vi "HFRR ADV v11.vi"() -> ()   [LabVIEW 2025] (continued)
        n1007 = property on="Imaging" class="Bool (strict)"("DisabledEnum"=w968) -> ()  [unwired: 2 in, 2 out]
        n1008 = property on="Analysis" class="Bool (strict)"("DisabledEnum"=w968) -> ()  [unwired: 2 in, 2 out]
        n1009 = property on="Home" class="Bool (strict)"("DisabledEnum"=w968) -> ()  [unwired: 2 in, 2 out]
        n1010 = property on="Report" class="Bool (strict)"("DisabledEnum"=w968) -> ()  [unwired: 2 in, 2 out]
        n1011 = property on="Test Setup" class="Bool (strict)"("DisabledEnum"=w968) -> ()  [unwired: 2 in, 2 out]
        n1012 = case shown="True" w967 {
          tunnel: [T16."Disabled" ("Disabled") T16."Enabled" ("Disabled")] -> w966
          frame False {
          }
          frame True {
          }
        }
        n1013 = property on="About" class="Bool (strict)"("DisabledEnum"=w966) -> ()  [unwired: 2 in, 2 out]
      }
      frame "Adv Scar" {
        w975 = T16."Enabled" ("Disabled")
        n1014 = property on="Dashboard" class="Bool (strict)"("DisabledEnum"=T16."Disabled" ("Disabled")) -> ()  [unwired: 2 in, 2 out]
        n1015 = property on="Imaging" class="Bool (strict)"("DisabledEnum"=w975) -> ()  [unwired: 2 in, 2 out]
        n1016 = property on="Analysis" class="Bool (strict)"("DisabledEnum"=w975) -> ()  [unwired: 2 in, 2 out]
        n1017 = property on="Home" class="Bool (strict)"("DisabledEnum"=w975) -> ()  [unwired: 2 in, 2 out]
        n1018 = property on="Report" class="Bool (strict)"("DisabledEnum"=w975) -> ()  [unwired: 2 in, 2 out]
        n1019 = property on="Test Setup" class="Bool (strict)"("DisabledEnum"=w975) -> ()  [unwired: 2 in, 2 out]
        n1020 = local read "Service Password enable"() -> (w973:bool)
        n1021 = case shown="True" w973 {
          tunnel: [T16."Disabled" ("Disabled") T16."Enabled" ("Disabled")] -> w972
          frame False {
          }
          frame True {
          }
        }
        n1022 = property on="About" class="Bool (strict)"("DisabledEnum"=w972) -> ()  [unwired: 2 in, 2 out]
      }
      frame "Adv Scar Report" {
        w980 = T16."Enabled" ("Disabled")
        n1023 = property on="Dashboard" class="Bool (strict)"("DisabledEnum"=T16."Disabled" ("Disabled")) -> ()  [unwired: 2 in, 2 out]
        n1024 = property on="Imaging" class="Bool (strict)"("DisabledEnum"=w980) -> ()  [unwired: 2 in, 2 out]
        n1025 = property on="Analysis" class="Bool (strict)"("DisabledEnum"=w980) -> ()  [unwired: 2 in, 2 out]
        n1026 = property on="Home" class="Bool (strict)"("DisabledEnum"=w980) -> ()  [unwired: 2 in, 2 out]
        n1027 = property on="Report" class="Bool (strict)"("DisabledEnum"=w980) -> ()  [unwired: 2 in, 2 out]
        n1028 = property on="Test Setup" class="Bool (strict)"("DisabledEnum"=w980) -> ()  [unwired: 2 in, 2 out]
        n1029 = local read "Service Password enable"() -> (w979:bool)
        n1030 = case shown="True" w979 {
          tunnel: [T16."Disabled" ("Disabled") T16."Enabled" ("Disabled")] -> w978
          frame False {
          }
          frame True {
          }
        }
        n1031 = property on="About" class="Bool (strict)"("DisabledEnum"=w978) -> ()  [unwired: 2 in, 2 out]
      }
      frame "Compare Files" {
        w986 = T16."Enabled" ("Disabled")
        n1032 = local read "Service Password enable"() -> (w985:bool)
        n1033 = property on="Dashboard" class="Bool (strict)"("DisabledEnum"=T16."Disabled" ("Disabled")) -> ()  [unwired: 2 in, 2 out]
        n1034 = property on="Imaging" class="Bool (strict)"("DisabledEnum"=w986) -> ()  [unwired: 2 in, 2 out]
        n1035 = property on="Analysis" class="Bool (strict)"("DisabledEnum"=w986) -> ()  [unwired: 2 in, 2 out]
        n1036 = property on="Home" class="Bool (strict)"("DisabledEnum"=w986) -> ()  [unwired: 2 in, 2 out]
        n1037 = property on="Report" class="Bool (strict)"("DisabledEnum"=w986) -> ()  [unwired: 2 in, 2 out]
        n1038 = property on="Test Setup" class="Bool (strict)"("DisabledEnum"=w986) -> ()  [unwired: 2 in, 2 out]
        n1039 = case shown="True" w985 {
          tunnel: [T16."Disabled" ("Disabled") T16."Enabled" ("Disabled")] -> w984
          frame False {
          }
          frame True {
          }
        }
        n1040 = property on="About" class="Bool (strict)"("DisabledEnum"=w984) -> ()  [unwired: 2 in, 2 out]
      }
      frame "Acquire" {
        n1041 = local read "Service Password enable"() -> (w990:bool)
        n1042 = property on="Test Setup" class="Bool (strict)"("DisabledEnum"=T16."Disabled" ("Disabled")) -> ()  [unwired: 2 in, 2 out]
        n1043 = local read "Auto Start Test"() -> (w992:bool)
        n1044 = local read "RUN"() -> (w994:bool)
        n1045 = case shown="True" w990 {
          tunnel: [T16."Disabled" ("Disabled") T16."Enabled" ("Disabled")] -> w991
          frame False {
          }
          frame True {
          }
        }
        n1046 = Or(x=w994, y=w992) -> (x .or. y?=w993:bool)
        n1047 = case shown="True" w993 {
          tunnel: [T16."Enabled" ("Disabled") T16."Disabled" ("Disabled")] -> w996
          frame False {
          }
          frame True {
          }
        }
        n1048 = property on="About" class="Bool (strict)"("DisabledEnum"=w991) -> ()  [unwired: 2 in, 2 out]
        n1049 = property on="Imaging" class="Bool (strict)"("DisabledEnum"=w996) -> ()  [unwired: 2 in, 2 out]
        n1050 = property on="Dashboard" class="Bool (strict)"("DisabledEnum"=w996) -> ()  [unwired: 2 in, 2 out]
        n1051 = property on="Analysis" class="Bool (strict)"("DisabledEnum"=w996) -> ()  [unwired: 2 in, 2 out]
        n1052 = property on="Home" class="Bool (strict)"("DisabledEnum"=w996) -> ()  [unwired: 2 in, 2 out]
        n1053 = property on="Report" class="Bool (strict)"("DisabledEnum"=w996) -> ()  [unwired: 2 in, 2 out]
      }
      frame "About" {
        n1054 = local read "FILE"() -> (w1009:string)
        n1055 = local read "TEST FILE NAM,E SAVED"() -> (w1002:bool)
        n1056 = call <vilib>:"Trim Whitespace.vi"("string"=w1009) -> ("trimmed string"=w1008:string)  [unwired: 1 in]
        n1057 = local read "Auto Start Test"() -> (w1012:bool)
        n1058 = String Length(string=w1008) -> (length=w1007:i32)
        n1059 = Greater?(x=w1007, y=1) -> (0:w1004:bool)
        n1060 = And(x=w1004, y=w1002) -> (x .and. y?=w1003:bool)
        n1061 = local read "RUN"() -> (w1014:bool)
        n1062 = case shown="True" w1003 {
          tunnel: [T16."Disabled" ("Disabled") T16."Enabled" ("Disabled")] -> w1005
          frame False {
          }
          frame True {
          }
        }
        n1063 = Or(x=w1014, y=w1012) -> (x .or. y?=w1013:bool)
        n1064 = property on="About" class="Bool (strict)"("DisabledEnum"=T16."Enabled" ("Disabled")) -> ()  [unwired: 2 in, 2 out]
        n1065 = case shown="False" w1013 {
          tunnel: [T16."Enabled" ("Disabled") T16."Disabled" ("Disabled")] -> w1011
          frame False {
          }
          frame True {
          }
        }
        n1066 = property on="Dashboard" class="Bool (strict)"("DisabledEnum"=w1005) -> ()  [unwired: 2 in, 2 out]
        n1067 = property on="Test Setup" class="Bool (strict)"("DisabledEnum"=T16."Disabled" ("Disabled")) -> ()  [unwired: 2 in, 2 out]
        n1068 = property on="Imaging" class="Bool (strict)"("DisabledEnum"=w1011) -> ()  [unwired: 2 in, 2 out]
        n1069 = property on="Analysis" class="Bool (strict)"("DisabledEnum"=w1011) -> ()  [unwired: 2 in, 2 out]
        n1070 = property on="Home" class="Bool (strict)"("DisabledEnum"=w1011) -> ()  [unwired: 2 in, 2 out]
        n1071 = property on="Report" class="Bool (strict)"("DisabledEnum"=w1011) -> ()  [unwired: 2 in, 2 out]
      }
    }
    n1072 = local read "Quit"() -> (w945:bool)
    "Single" <- "Single - Graph"
  }
  n1073 = disable-structure shown="Disabled" {
    disable-tunnel: [w1280 _] -> w36
    disable-tunnel: _ -> [w1279 _]
    frame Disabled {
      n1074 = while {
        tunnel: w1279 -> [_]
        tunnel: [w1281] -> w1280
        tunnel: [w1282] -> _
        i -> [w1282]
        stop <- w1281 stop-if-true
        w1298 = u16 10 items=["1.0"=10, "1.5"=15, "2.0"=20] ("stop bits (10: 1 bit)")
        n1075 = Wait (ms)(milliseconds to wait=u32 10) -> ()  [unwired: 1 out]
        n1076 = call-poly "VISA Configure Serial Port"("VISA resource name"=refnum<visa-resource-name> "ASRL1::INSTR" ("COM PORT"), "timeout (10sec)"=u32 10, "baud rate (9600)"=u32 57600, "data bits (8)"=u16 8, "stop bits (10: 1 bit)"=w1298) -> ("VISA resource name out"=w1284:refnum<visa-resource-name>, "error out"=w1293:errorcluster)  [unwired: 9 in]
        n1077 = VISA Read(VISA resource name=w1284, byte count=u32 2 ("byte count (0)")) -> (read buffer=w1292:string)  [unwired: 1 in, 3 out]
        n1078 = String Subset(string=w1292, offset (0)=0, length (rest)=2 ("length (rest)")) -> (substring=w1291:string)
        n1079 = Match Pattern(string=w1291, regular expression="<>") -> (offset past match=w1288:i32)  [unwired: 1 in, 3 out]
        n1080 = Greater Or Equal?(x=w1288, y=0) -> (x >= y?=w1283:bool)
        n1081 = case shown="True" w1283 {
          tunnel: w1284 -> [_ w1302]
          tunnel: w1293 -> [_ w1301]
          frame False {
          }
          frame True {
            n1082 = VISA Read(VISA resource name=w1302, byte count=u32 32 ("byte count (0)"), error in (no error)=w1301) -> (read buffer=w1300:string)  [unwired: 3 out]
            n1083 = String Subset(string=w1300, offset (0)=0, length (rest)=8 ("length (rest)")) -> (substring=w1304:string)
            n1084 = String Subset(string=w1300, offset (0)=8, length (rest)=8 ("length (rest)")) -> (substring=w1305:string)
            n1085 = Decimal String To Number(string=w1305) -> (number=w1312:i32)  [unwired: 2 in, 1 out]
            n1086 = Decimal String To Number(string=w1304) -> (number=w1308:i32)  [unwired: 2 in, 1 out]
            n1087 = Divide(x=w1312, y=10000) -> ()  [unwired: 1 out]
            n1088 = Divide(x=w1308, y=1000000) -> ()  [unwired: 1 out]
          }
        }
        n1089 = local read "Quit"() -> (w1281:bool)
      }
    }
    frame Enabled {
    }
  }
  n1090 = local write "Err Count"(0 ("Err Count")) -> ()
  n1091 = local write "FRICVALZ"(0.0 ("FRICVALZ")) -> ()
  n1092 = Tick Count (ms)() -> (millisecond timer value=w49:u32)
  n1093 = while {
    shift-right: [w1331] -> w53
    shift-left: _ -> [w1320]
    shift-right: [w1330] -> w52
    shift-left: errorcluster {"status"=TRUE, "code"=0, "source"="Init"} ("error IO") -> [w1322]
    shift-right: [w1328] -> _
    shift-left: w49 -> [w1329]
    tunnel: [w1315] -> w40
    tunnel: [w1327] -> _
    i -> [w1327]
    stop <- w1315 stop-if-true
    n1094 = local read "Com Port 1"() -> (w1321:refnum<visa-resource-name>)
    n1095 = local read "Port 1a"() -> (w1323:bool)
    n1096 = local read "Port 3"() -> (w1324:bool)
    n1097 = Not Equal?(x=w1321, y=w1320) -> (x != y?=w1319:bool)
    n1098 = Or(x=w1324, y=w1323) -> (x .or. y?=w1326:bool)
    n1099 = Unbundle(w1322) -> ("status"=→"Port 3":bool)  [unwired: 2 out]
    n1100 = flat-sequence {
      tunnel: [w1334] -> w1318
      tunnel: w1322 -> [w1334]
      frame #0 {
        n1101 = Wait (ms)(milliseconds to wait=u32 200) -> ()  [unwired: 1 out]
      }
    }
    n1102 = case shown="True" w1326 {
      frame False {
        w1336 = FALSE ("Visible")
        n1103 = property on="Port 1a" class="Bool (strict)"("Visible"=w1336) -> ()  [unwired: 2 in, 2 out]
        n1104 = property on="Port 3" class="Bool (strict)"("Visible"=w1336) -> ()  [unwired: 2 in, 2 out]
      }
      frame True {
        w1337 = TRUE ("Visible")
        n1105 = property on="Port 1a" class="Bool (strict)"("Visible"=w1337) -> ()  [unwired: 2 in, 2 out]
        n1106 = property on="Port 3" class="Bool (strict)"("Visible"=w1337) -> ()  [unwired: 2 in, 2 out]
      }
    }
    n1107 = Or(x=w1319, y="Re-initialize Port1") -> (x .or. y?=w1316:bool)
    n1108 = case shown="True" w1316 {
      tunnel: [w1332 errorcluster {"status"=TRUE, "code"=0, "source"="Init"} ("error out")] -> w1317
      tunnel: w1318 -> [w1332 _]
      frame False {
      }
      frame True {
      }
    }
    n1109 = case shown="No Error" w1317 {
      selector: w1317 -> [w1338 w1683]
      tunnel: [w1343 w1688] -> w1331
      tunnel: [w1342 w1680] -> w1330
      tunnel: w1320 -> [w1341 w1686]
      tunnel: w1329 -> [w1340 w1685]
      tunnel: [w1339 w1685] -> w1328
      frame No Error {
        n1110 = stacked-sequence {
          tunnel: [w1353 _ _ _ _ _] -> w1343
          tunnel: [w1352 _ _ _ _ _] -> w1342
          tunnel: w1341 -> [w1348 _ _ _ _ _]
          tunnel: w1338 -> [w1347 _ _ _ _ _]
          tunnel: w1340 -> [_ w1476 _ _ _ _]
          tunnel: [_ w1475 _ _ _ _] -> w1339
          tunnel: [_ w1447 _ _ _ _] -> _
          frame #0 {
            n1111 = property class="Instr"(reference=w1348, error in=w1347) -> (reference out=w1350:refnum<visa-resource-name>, error out=w1351:errorcluster, "Serial Settings:Number of Bytes at Serial Port"=w1344:u32)
            "Sps 3" <- w1344
            "Port 1" <- w1344
            n1112 = Greater?(x=w1344, y=u32 5) -> (0:w1346:bool)
            n1113 = case shown="True" w1346 {
              tunnel: w1350 -> [w1355 w1382]
              tunnel: w1351 -> [w1354 w1361]
              tunnel: [w1354 w1357] -> w1352
              tunnel: [w1355 w1383] -> w1353
              frame False {
              }
              frame True {
                w1356 = TRUE ("PAUSE")
                w1359 = TRUE ("PAUSE")
                # "Out as Volts"
                n1114 = call "ELAPSED TIMER VI - uno.vi"("error in"=w1361, "RESET"=w1359, "PAUSE"=w1359) -> ("error out"=w1360:errorcluster)  [unwired: 6 in, 2 out]
                n1115 = local read "Residual Uno"() -> (w1376:string)
                n1116 = while {
                  tunnel: [w1431] -> w1358
                  tunnel: [w1430] -> w1383
                  tunnel: w1360 -> [w1429]
                  tunnel: w1382 -> [w1428]
                  tunnel: [w1425] -> _
                  shift-right: [w1421] -> w1364
                  shift-left: w1376 -> [w1423]
                  i -> [w1425]
                  stop <- w1420 stop-if-true
                  w1418 = FALSE ("PAUSE")
                  n1117 = property class="Instr"(reference=w1428, error in=w1429) -> (reference out=w1433:refnum<visa-resource-name>, error out=w1432:errorcluster, "Serial Settings:Number of Bytes at Serial Port"=w1424:u32)
                  n1118 = local read "Quit"() -> (w1419:bool)
                  n1119 = call "ELAPSED TIMER VI - uno.vi"("TARGET"=5.0, "RESET"=w1418, "PAUSE"=w1418) -> ("ELAPSED INDICATION"=w1416:bool)  [unwired: 6 in, 2 out]
                  "ELAPSED INDICATION" <- w1416
                  n1120 = VISA Read(VISA resource name=w1433, byte count=w1424, error in (no error)=w1432) -> (VISA resource name out=w1430:refnum<visa-resource-name>, read buffer=w1422:string, error out=w1431:errorcluster)  [unwired: 1 out]
                  n1121 = Greater?(x=w1424, y=u32 30) -> (0:w1426:bool)
                  n1122 = Concatenate Strings(w1423, w1422) -> (w1421:string)
                  n1123 = Compound Arithmetic op=OR(w1426, w1419, w1416) -> (w1420:bool)
                }
                "UnoRead" <- w1364
                n1124 = call "ELAPSED TIMER VI - uno.vi"("error in"=w1358, "RESET"=w1356, "PAUSE"=w1356) -> ("error out"=w1357:errorcluster)  [unwired: 6 in, 2 out]
                n1125 = while {
                  shift-right: [w1402] -> w1375
                  shift-left: w1364 -> [w1408]
                  tunnel: [w1401] -> w1371 mode=indexing
                  tunnel: [w1403] -> _
                  i -> [w1403]
                  stop <- w1400 stop-if-true
                  n1126 = Match Pattern(string=w1408, regular expression="*") -> (after substring=w1406:string)  [unwired: 1 in, 3 out]
                  n1127 = local read "Quit"() -> (w1399:bool)
                  n1128 = local read "ELAPSED INDICATION"() -> (w1398:bool)
                  n1129 = Match Pattern(string=w1406, regular expression="&") -> (before substring=w1401:string, after substring=w1402:string, offset past match=w1404:i32)  [unwired: 1 in, 1 out]
                  n1130 = Less Than 0?(x=w1404) -> (x < 0?=w1405:bool)
                  n1131 = Compound Arithmetic op=OR(w1405, w1399, w1398) -> (w1400:bool)
                }
                n1132 = local write "Residual Uno"(w1375) -> ()
                n1133 = Array Size(array=w1371) -> (size(s)=w1372:i32)
                n1134 = Decrement(x=w1372) -> (x-1=w1374:i32)
                n1135 = Delete From Array(array=w1371, length=1, index=w1374) -> (array with subset deleted=w1369:string[])  [unwired: 1 out]
                n1136 = Array Size(array=w1369) -> (size(s)=w1368:i32)
                n1137 = Decrement(x=w1368) -> (x-1=w1367:i32)
                n1138 = while {
                  tunnel: [w1397] -> w1380 mode=indexing
                  tunnel: [w1396] -> w1379 mode=indexing
                  tunnel: w1369 -> [w1390] mode=indexing
                  tunnel: w1367 -> [w1389]
                  tunnel: [w1388] -> _
                  i -> [w1388]
                  stop <- w1384 stop-if-true
                  w1391 = 0 ("length (rest)")
                  w1393 = ";" ("regular expression")
                  n1139 = local read "ELAPSED INDICATION"() -> (w1387:bool)
                  n1140 = Less Or Equal?(x=w1389, y=w1388) -> (x <= y?=w1385:bool)
                  n1141 = local read "Quit"() -> (w1386:bool)
                  n1142 = Compound Arithmetic op=OR(w1385, w1386, w1387) -> (w1384:bool)
                  n1143 = Match Pattern(string=w1390, regular expression=w1393) -> (before substring=w1395:string, after substring=w1394:string)  [unwired: 1 in, 2 out]
                  n1144 = Decimal String To Number(string=w1395, default (0L)=w1391) -> (number=w1397:i32)  [unwired: 1 in, 1 out]
                  n1145 = Match Pattern(string=w1394, regular expression=w1393) -> (before substring=w1392:string)  [unwired: 1 in, 3 out]
                  n1146 = Decimal String To Number(string=w1392, default (0L)=w1391) -> (number=w1396:i32)  [unwired: 1 in, 1 out]
                }
                n1147 = case shown="0, Default" "ADC Res" {
                  tunnel: [w1411 w1413] -> w1363
                  frame 0, Default {
                    n1148 = Divide(x=65535 ("length (rest)"), y=2 ("length (rest)")) -> (x/y=w1411:dbl)
                  }
                  frame 1 {
                    n1149 = Divide(x=16777216 ("length (rest)"), y=2 ("length (rest)")) -> (x/y=w1413:dbl)
                  }
                }
                n1150 = Bundle(w1380, w1379) -> (w1370:cluster{i32[], i32[]})  [unwired: 1 in]
                n1151 = Divide(x=w1370, y=w1363) -> (x/y=w1381:cluster{dbl[], dbl[]})
                n1152 = Multiply(x=w1381, y=sgl 5.03 ("Numeric")) -> (x*y=w1378:cluster{dbl[], dbl[]})
                n1153 = Unbundle(w1378) -> (→"Ch1":dbl[], →"Ch0":dbl[])
              }
            }
            n1154 = Not(x=w1346) -> (.not. x?=→"Port 1a":bool)
          }
          frame #1 {
            n1155 = local read "zOff 2"() -> (w1468:dbl)
            n1156 = local read "Ch1"() -> (w1458:dbl[])
            n1157 = case shown="True" "Zero 2" {
              tunnel: w1458 -> [_ w1488]
              frame False {
              }
              frame True {
                n1158 = call-poly <vilib>:"Mean.vi"("X"=w1488) -> ("mean"=→"zOff 2":dbl)  [unwired: 1 out]
                n1159 = local write "Zero 2"(FALSE ("Zero")) -> ()
              }
            }
            n1160 = Subtract(x=w1458, y=w1468) -> (x-y=w1464:dbl[])
            n1161 = call-poly <vilib>:"Mean.vi"("X"=w1458) -> ("mean"=w1459:dbl)  [unwired: 1 out]
            "Slide 3" <- w1459
            n1162 = Multiply(x=w1464, y=1.0 ("PG Oth")) -> (x*y=w1450:dbl[])
            n1163 = local read "FF buffer"() -> (w1455:dbl[])
            n1164 = Divide(x=w1450, y=1) -> (x/y=w1449:dbl[])
            "Fric Val" <- w1449
            n1165 = call <vilib>:"Mean PtByPt.vi"("x"=w1459, "sample length"=10, "initialize"="Reset 2") -> ("mean"=→"Mean Pos Fil 2":dbl)  [unwired: 1 in, 1 out]
            n1166 = Array Size(array=w1455) -> (size(s)=w1457:i32)
            n1167 = call-poly <vilib>:"Mean.vi"("X"=w1449) -> ("mean"=w1463:dbl)  [unwired: 1 out]
            n1168 = Insert Into Array(array=w1455, index=w1457, new element=w1449) -> (w1452:dbl[])
            n1169 = Array Size(array=w1452) -> (size(s)=w1451:i32)
            n1170 = case shown="True" "DC corr 2" {
              tunnel: w1449 -> [w1491 w1494]
              tunnel: [w1491 w1493] -> w1456
              tunnel: w1463 -> [_ w1492]
              frame False {
              }
              frame True {
                n1171 = Subtract(x=w1494, y=w1492) -> (x-y=w1493:dbl[])
              }
            }
            n1172 = Tick Count (ms)() -> (millisecond timer value=w1475:u32)
            n1173 = Greater?(x=w1451, y=1000) -> (0:w1453:bool)
            n1174 = Subtract(x=w1475, y=w1476) -> (x-y=w1474:u32)
            n1175 = case shown="True" w1453 {
              tunnel: [w1481 w1484] -> w1440
              tunnel: w1452 -> [w1481 w1487]
              tunnel: w1451 -> [_ w1486]
              frame False {
              }
              frame True {
                n1176 = Subtract(x=w1486, y=1000) -> (x-y=w1482:i32)
                n1177 = Delete From Array(array=w1487, length=w1482, index=0) -> (array with subset deleted=w1484:dbl[])  [unwired: 1 out]
              }
            }
            n1178 = Divide(x=w1474, y=u32 1000 ("x")) -> (x/y=w1472:dbl)
            n1179 = Array Size(array=w1456) -> (size(s)=w1471:i32)
            n1180 = Divide(x=w1471, y=w1472) -> (x/y=w1467:dbl)
            "Sps 2" <- w1467
            n1181 = Reciprocal(x=w1467) -> (1/x=w1465:dbl)
            "dt" <- w1465
            n1182 = local read "FRIC. FORCE :"() -> (w1437:dbl)
            n1183 = local write "FF buffer"(w1440) -> ()
            n1184 = Negate(x=w1440) -> (-x=w1439:dbl[])
            n1185 = call "Elapsed Time5"("Time Target (s)"="check time s", "Reset"="Reset 3") -> ("Time has Elapsed"=w1442:bool)  [unwired: 10 in, 7 out]
            n1186 = Array Max & Min(array=w1439) -> (max value=w1447:dbl)  [unwired: 3 out]
            n1187 = Bundle By Name("Y"=w1456, "dt"=w1465, "t0"=timestamp(0 s since 1904-01-01)) -> (w1435:waveform(dbl))  [unwired: 1 in]
            n1188 = Multiply(x=w1437, y=21.1986) -> (x*y=w1436:dbl)
            n1189 = Greater Or Equal?(x=w1447, y="Threshold value") -> (x >= y?=w1443:bool)
            n1190 = Multiply(x=w1436, y=w1435) -> (x*y=→"FF_Wfm":waveform(dbl))
            n1191 = And(x=w1443, y=w1442) -> (x .and. y?=w1441:bool)
            n1192 = case shown="True" w1441 {
              frame False {
                n1193 = local write "Reset 3"(FALSE ("Reset 3")) -> ()
              }
              frame True {
                n1194 = local write "Reset 3"(TRUE ("Reset 3")) -> ()
                n1195 = local write "save dpt"(TRUE ("save dpt")) -> ()
              }
            }
          }
          frame #2 {
            n1196 = local read "FF buffer"() -> (w1501:dbl[])
            n1197 = Array Max & Min(array=w1501) -> (max value=w1496:dbl, min value=w1497:dbl)  [unwired: 2 out]
            n1198 = Subtract(x=w1496, y=w1497) -> (x-y=w1498:dbl)
            n1199 = Multiply(x=1.0 ("y 2"), y="Threshold") -> ()  [unwired: 1 out]
            n1200 = Greater?(x=w1498, y="Threshold") -> (0:w1495:bool)
            n1201 = case shown="True" w1495 {
              tunnel: w1501 -> [_ w1508]
              tunnel: [_ w1506] -> _
              frame False {
              }
              frame True {
                w1507 = 1.0 ("y")
                n1202 = Delete From Array(array=w1508, length=100, index=0) -> (deleted portion=w1513:dbl[])  [unwired: 1 out]
                n1203 = call-poly <vilib>:"Mean.vi"("X"=w1513) -> ("mean"=w1512:dbl)  [unwired: 1 out]
                n1204 = Subtract(x=w1508, y=w1512) -> (x-y=w1511:dbl[])
                n1205 = Multiply(x=w1507, y=w1507) -> (x*y=w1509:dbl)
                n1206 = Multiply(x=w1511, y=w1509) -> (x*y=w1510:dbl[])
                "FF cal val" <- w1510
                n1207 = Array Size(array=w1510) -> (size(s)=w1504:i32)
                n1208 = Array Max & Min(array=w1510) -> (max value=w1503:dbl, min value=w1502:dbl)  [unwired: 2 out]
                n1209 = property on="FF Calibration g" class="WFGraph (strict)"("X Scale.Range:Minimum"=0.0 ("y"), "X Scale.Range:Maximum"=w1504, "Y Scale.Range:Minimum"=w1503, "Y Scale.Range:Maximum"=w1502) -> ()  [unwired: 2 in, 2 out]
                n1210 = local read "FRIC. FORCE :"() -> (w1506:dbl)
              }
            }
          }
          frame #3 {
            # "5"
            n1211 = local read "DISPLACEMENT :"() -> (w1604:dbl)
            n1212 = Multiply(x=w1604, y=1.0) -> (x*y=w1522:dbl)
            n1213 = local read "zOff 3"() -> (w1607:dbl)
            n1214 = local read "Ch0"() -> (w1535:dbl[])
            n1215 = case shown="True" "Zero 3" {
              tunnel: w1535 -> [_ w1622]
              frame False {
              }
              frame True {
                n1216 = call-poly <vilib>:"Mean.vi"("X"=w1622) -> ("mean"=→"zOff 3":dbl)  [unwired: 1 out]
                n1217 = local write "Zero 3"(FALSE ("Zero")) -> ()
              }
            }
            n1218 = Add(x=w1535, y="Offset") -> (x+y=w1534:dbl[])
            n1219 = Multiply(x=w1522, y="DISPLACEMENT : 2") -> (x*y=w1589:dbl)
            n1220 = Subtract(x=w1535, y=w1607) -> (x-y=w1592:dbl[])
            n1221 = Multiply(x=w1592, y=w1589) -> (x*y=w1591:dbl[])
            n1222 = Multiply(x=w1592, y=w1522) -> (x*y=w1603:dbl[])
            "ABS DP" <- w1603
            n1223 = local read "Standard Slip Gauge (mm)"() -> (w1590:dbl)
            n1224 = call-poly <vilib>:"Mean.vi"("X"=w1591) -> ("mean"=w1521:dbl)  [unwired: 1 out]
            "Disp (mm)" <- w1521
            "software msrnt" <- w1521
            n1225 = Multiply(x=w1534, y="Gain") -> (x*y=w1529:dbl[])
            "Voltage LVDT Acq" <- w1529
            "gLVDTraw" <- w1529
            n1226 = call-poly <vilib>:"Mean.vi"("X"=w1603) -> ("mean"=w1594:dbl)  [unwired: 1 out]
            n1227 = case shown="True" "DC correction" {
              tunnel: w1603 -> [w1625 w1628]
              tunnel: [w1625 w1627] -> w1541
              tunnel: w1594 -> [_ w1626]
              frame False {
              }
              frame True {
                n1228 = Subtract(x=w1628, y=w1626) -> (x-y=w1627:dbl[])
              }
            }
            n1229 = Divide(x=w1521, y=w1590) -> (x/y=w1588:dbl)
            n1230 = call-poly <vilib>:"Mean.vi"("X"=w1529) -> ("mean"=w1528:dbl)  [unwired: 1 out]
            n1231 = Array Max & Min(array=w1529) -> (max value=w1533:dbl, min value=w1532:dbl)  [unwired: 2 out]
            n1232 = Multiply(x=w1588, y=w1589) -> (x*y=→"DISPLACEMENT : 3":dbl)
            n1233 = Subtract(x=w1533, y=w1532) -> (x-y=→"Pk-Pk":dbl)
            n1234 = local read "dt"() -> (w1606:dbl)
            n1235 = Threshold 1D Array(2:0.0 ("threshold y"), 3:w1541) -> (0:w1558:dbl)  [unwired: 1 in]
            n1236 = Bundle By Name("Y"=w1541, "dt"=w1606, "t0"=timestamp(0 s since 1904-01-01)) -> (w1596:waveform(dbl))  [unwired: 1 in]
            n1237 = local read "FF_Wfm"() -> (w1595:waveform(dbl))
            n1238 = Equal To 0?(x=w1558) -> (x = 0?=w1559:bool)
            n1239 = case shown="True" w1559 {
              tunnel: w1541 -> [_ w1616]
              tunnel: [w1612 w1613] -> w1554
              tunnel: w1558 -> [w1612 _]
              frame False {
              }
              frame True {
                n1240 = Threshold 1D Array(1:20 ("start index (0)"), 2:0.0 ("threshold y"), 3:w1616) -> (0:w1613:dbl)
              }
            }
            n1241 = Build Array(w1596, w1595) -> (w1577:waveform(dbl)[])
            "Waveform Graph 2" <- w1577
            n1242 = call-poly <vilib>:"Extract Single Tone Information.vi"("time signal in"=w1596) -> ("detected amplitude"=w1530:dbl, "detected frequency"=→"RawFreq":dbl)  [unwired: 5 in, 4 out]
            n1243 = Multiply(x=w1530, y=2.0) -> (x*y=w1517:dbl)
            n1244 = Subtract(x=w1528, y="LvdtOff") -> (x-y=w1527:dbl)
            n1245 = local read "StrokeL"() -> (w1518:dbl)
            n1246 = Not A Number/Path/Refnum?(number/path/refnum=w1517) -> (NaN/Path/Refnum?=w1519:bool)
            n1247 = Subtract(x=w1527, y=w1530) -> (x-y=w1539:dbl)
            n1248 = Add(x=w1530, y=w1527) -> (x+y=w1538:dbl)
            n1249 = Index Array(array=w1577) -> (element #1=w1578:waveform(dbl), element #2=w1580:waveform(dbl))  [unwired: 2 in]
            n1250 = Select(t=w1518, s=w1519, f=w1517) -> (s? t:f=w1516:dbl)
            "Stroke" <- w1516
            "Mean(RAW) Stroke" <- w1516
            "StrokeL" <- w1516
            n1251 = Bundle(w1527, w1539, w1538) -> (→"Slide 8":cluster{dbl, dbl, dbl})  [unwired: 1 in]
            n1252 = Unbundle By Name(w1578) -> ("Y"=w1551:dbl[])
            n1253 = Split 1D Array(array=w1541, index=w1554) -> (second subarray=w1555:dbl[])  [unwired: 1 out]
            n1254 = In Range and Coerce(upper limit=1.5, x=w1516, lower limit=0.5) -> (In Range?=w1600:bool)  [unwired: 1 out]
            n1255 = Split 1D Array(array=w1551, index="Window") -> (second subarray=w1569:dbl[])  [unwired: 1 out]
            n1256 = Unbundle By Name(w1580) -> ("Y"=w1552:dbl[])
            n1257 = Threshold 1D Array(1:180 ("start index (0)"), 2:0.0 ("threshold y"), 3:w1555) -> (0:w1553:dbl)
            n1258 = local read "Test \nStatus"() -> (w1597:bool)
            n1259 = Split 1D Array(array=w1552, index=w1554) -> (second subarray=w1549:dbl[])  [unwired: 1 out]
            n1260 = Not(x=w1600) -> (.not. x?=w1599:bool)
            n1261 = call-poly <vilib>:"RMS.vi"("X"=w1569) -> ("rms value"=w1525:dbl)  [unwired: 1 out]
            "Current (A)" <- w1525
            n1262 = Array Max & Min(array=w1569) -> (max value=w1583:dbl, min value=w1584:dbl)  [unwired: 2 out]
            n1263 = Array Max & Min(array=w1552) -> (max value=w1581:dbl, min value=w1582:dbl)  [unwired: 2 out]
            n1264 = Subtract(x=w1583, y=w1584) -> (x-y=w1585:dbl)
            n1265 = Subtract(x=w1581, y=w1582) -> (x-y=w1586:dbl)
            n1266 = And(x=w1599, y=w1597) -> (x .and. y?=w1598:bool)
            n1267 = Split 1D Array(array=w1555, index=w1553) -> (first subarray=w1548:dbl[])  [unwired: 1 out]
            n1268 = Split 1D Array(array=w1549, index=w1553) -> (first subarray=w1546:dbl[])  [unwired: 1 out]
            n1269 = case shown="True" w1598 {
              tunnel: [i32[] [] w1618] -> _
              frame False {
              }
              frame True {
                n1270 = local read "UnoRead"() -> (w1620:string)
                n1271 = local read "Array"() -> (w1621:string[])
                n1272 = Build Array (concatenate)(w1621, w1620) -> (w1619:string[])
                "Array" <- w1619
                n1273 = String Length(string=w1619) -> (length=w1618:i32[])
              }
            }
            n1274 = local read "G_val"() -> (w1571:dbl)
            n1275 = Divide(x=w1586, y=w1585) -> (x/y=w1574:dbl)
            n1276 = call-poly <vilib>:"RMS.vi"("X"=w1546) -> ("rms value"=w1570:dbl)  [unwired: 1 out]
            n1277 = call-poly <vilib>:"Hanning Window.vi"("X"=w1548) -> ("Windowed X"=w1547:dbl[])  [unwired: 1 out]
            n1278 = call-poly <vilib>:"Hanning Window.vi"("X"=w1546) -> ("Windowed X"=w1545:dbl[])  [unwired: 1 out]
            n1279 = local read "Constant (G)"() -> (w1563:dbl)
            n1280 = Divide(x=w1570, y=w1525) -> (x/y=w1564:dbl)
            n1281 = Build Array(w1547, w1545) -> (→"Waveform Graph 4":dbl[][])
            n1282 = Multiply(x=w1574, y=0.2) -> (x*y=w1576:dbl)
            n1283 = Multiply(x=0.8 ("y"), y=w1571) -> (x*y=w1575:dbl)
            n1284 = Add(x=w1576, y=w1575) -> (x+y=w1543:dbl)
            n1285 = Multiply(x=w1564, y=0.2) -> (x*y=w1565:dbl)
            n1286 = Multiply(x=0.8 ("y"), y=w1563) -> (x*y=w1566:dbl)
            n1287 = Add(x=w1565, y=w1566) -> (x+y=w1562:dbl)
            "Constant (G)" <- w1562
            n1288 = Not A Number/Path/Refnum?(number/path/refnum=w1543) -> (NaN/Path/Refnum?=w1542:bool)
            n1289 = Select(t=0.0, s=w1542, f=w1543) -> (s? t:f=w1523:dbl)
            "G_val" <- w1523
            n1290 = Multiply(x=w1525, y=w1523) -> (x*y=→"Friction Force (N)":dbl)
            n1291 = Bundle(w1562, "t"=w1523) -> (→"pk-pk":cluster{dbl, "t":dbl})  [unwired: 1 in]
          }
          frame #4 {
            # "C:\\WinDucom\\data\\"
            # "?C:\\LAB-IQ-NXT\\data"
            n1292 = case shown="True" "save dpt" {
              frame False {
              }
              frame True {
                n1293 = local write "save dpt"(FALSE ("Hold 3")) -> ()
                n1294 = local read "file count"() -> (w1632:i32)
                n1295 = Number To Decimal String(number=w1632) -> (decimal integer string=w1638:string)  [unwired: 1 in]
                n1296 = Add(x=1, y=w1632) -> (x+y=w1633:i32)
                n1297 = local write "file count"(w1633) -> ()
                n1298 = local read "FILE 2"() -> (w1637:string)
                n1299 = Concatenate Strings(w1637, w1638) -> (w1630:string)
                n1300 = Concatenate Strings("C:\\LAB-IQ\\data" ("Substring"), w1630) -> (w1645:string)
                n1301 = local read "FF buffer"() -> (w1640:dbl[])
                n1302 = local read "ABS DP"() -> (w1639:dbl[])
                n1303 = Concatenate Strings(w1645, ".dpf" ("Substring")) -> (w1643:string)
                n1304 = Build Array(w1640, w1639) -> (w1635:dbl[][])
                n1305 = Concatenate Strings("FF ( V ); DP( mincron ) " ("character string"), "\r") -> (w1649:string)
                n1306 = String To Path(string=w1643) -> (path=w1641:path)
                n1307 = Transpose 2D Array(2D array=w1635) -> (transposed array=w1634:dbl[][])
                n1308 = call <vilib>:"Write Characters To File.vi"("append to file? (new file:F)"=FALSE, "character string"=w1649, "file path (dialog if empty)"=w1641) -> ("new file path (Not A Path if cancelled)"=w1646:path)  [unwired: 2 in]
                n1309 = Array To Spreadsheet String(delimiter (Tab)=";", array=w1634, 3:"" ("format string")) -> (spreadsheet string=w1636:string)
                "String 9" <- w1636
                n1310 = call <vilib>:"Write Characters To File.vi"("append to file? (new file:F)"=TRUE, "character string"=w1636, "file path (dialog if empty)"=w1646) -> ()  [unwired: 2 in, 1 out]
              }
            }
          }
          frame #5 {
            n1311 = case shown="True" "Hold 4" {
              frame False {
              }
              frame True {
                n1312 = File Dialog(6:"*.dpf" ("pattern"), 11:path "C:/LAB-IQ" ("start path")) -> (0:w1656:errorcluster, 3:w1671:path)  [unwired: 5 in, 2 out]
                n1313 = Unbundle(w1656) -> ()  [unwired: 3 out]
                n1314 = call <vilib>:"Read Characters From File.vi"("file path (dialog if empty)"=w1671) -> ("character string"=w1661:string)  [unwired: 5 in, 3 out]
                n1315 = Spreadsheet String To Array(delimiter (Tab)=";", format string="%S", spreadsheet string=w1661, array type (2D Dbl)=string[][] []) -> (array=w1665:string[][])
                n1316 = for {
                  tunnel: w1665 -> [w1675] mode=indexing
                  tunnel: [w1674] -> w1666 mode=indexing
                  n1317 = for {
                    tunnel: w1675 -> [w1677] mode=indexing
                    tunnel: [w1676] -> w1674 mode=indexing
                    n1318 = call <vilib>:"Trim Whitespace.vi"("string"=w1677) -> ("trimmed string"=w1676:string)  [unwired: 1 in]
                  }
                }
                n1319 = Fract/Exp String To Number(string=w1666) -> (number=w1668:dbl[][])  [unwired: 3 in, 1 out]
                n1320 = Array Subset(array=w1668, index (row)=1 ("index (col)")) -> (w1670:dbl[][])  [unwired: 3 in]
                n1321 = Index Array(array=w1670, index (col) #1=0 ("disabled index (col)"), index (col) #2=1 ("disabled index (col)")) -> (element #1=w1659:dbl[], element #2=w1658:dbl[])  [unwired: 2 in]
                n1322 = Build Array(w1659, w1658) -> (→"Waveform Graph":dbl[][])
              }
            }
          }
        }
      }
      frame Error {
        w1694 = u16 0 items=["None", "XON/XOFF", "RTS/CTS", "XON/XOFF & RTS/CTS", "DTR/DSR", "XON/XOFF & DTR/DSR"] ("flow control (0:none)  2")
        w1692 = u16 10 items=["1.0"=10, "1.5"=15, "2.0"=20] ("stop bits 2")
        w1690 = u16 0 items=["None", "Odd", "Even", "Mark", "Space"] ("parity 2")
        w1691 = u32 10000  # timeout (10sec)
        n1323 = VISA Close(VISA resource name=w1686, error in (no error)=w1683) -> (error out=w1687:errorcluster)
        n1324 = local write "Sps 3"(0.0 ("Sps 4")) -> ()
        n1325 = local write "Port 1a"(FALSE ("Port 1a")) -> ()
        n1326 = call <vilib>:"Clear Errors.vi"("error in (no error)"=w1687) -> ("error out"=w1684:errorcluster)  [unwired: 5 in, 1 out]
        n1327 = local read "Com Port 1"() -> (w1679:refnum<visa-resource-name>)
        n1328 = call-poly "VISA Configure Serial Port"("VISA resource name"=w1679, "timeout (10sec)"=w1691, "baud rate (9600)"=u32 250000 ("baud rate  2"), "data bits (8)"=u16 8 ("data bits  2"), "parity (0:none)"=w1690, "error in (no error)"=w1684, "stop bits (10: 1 bit)"=w1692, "flow control (0:none)"=w1694) -> ("VISA resource name out"=w1695:refnum<visa-resource-name>, "error out"=w1696:errorcluster)  [unwired: 6 in]
        n1329 = flat-sequence {
          tunnel: w1695 -> [w1698]
          tunnel: w1696 -> [w1697]
          tunnel: [w1698] -> w1688
          tunnel: [w1697] -> w1680
          frame #0 {
            n1330 = Wait (ms)(milliseconds to wait=u32 50) -> ()  [unwired: 1 out]
          }
        }
        "Residual Uno" <- ""
        "Port 1 Error" <- w1680
      }
    }
    n1331 = local read "Quit"() -> (w1315:bool)
    "Error Uno" <- w1322
  }
  n1332 = while {
    shift-right: [w1715] -> w34
    shift-left: _ -> [w1706]
    shift-right: [w1714] -> w33
    shift-left: errorcluster {"status"=FALSE, "code"=0, "source"="Init"} ("error out") -> [w1708]
    tunnel: [w1701] -> w39
    tunnel: [w1713] -> _
    i -> [w1713]
    stop <- w1701 stop-if-true
    n1333 = local read "Com Port 2"() -> (w1707:refnum<visa-resource-name>)
    n1334 = local read "Port 2a"() -> (w1709:bool)
    n1335 = local read "Port 4"() -> (w1710:bool)
    n1336 = Not Equal?(x=w1707, y=w1706) -> (x != y?=w1705:bool)
    n1337 = Or(x=w1710, y=w1709) -> (x .or. y?=w1712:bool)
    n1338 = Unbundle(w1708) -> ("status"=→"Port 4":bool)  [unwired: 2 out]
    n1339 = flat-sequence {
      tunnel: w1708 -> [w1719]
      tunnel: [w1719] -> w1704
      frame #0 {
        n1340 = Wait (ms)(milliseconds to wait=u32 50) -> ()  [unwired: 1 out]
      }
    }
    n1341 = case shown="True" w1712 {
      frame False {
        w1720 = FALSE ("Visible")
        n1342 = property on="Port 2a" class="Bool (strict)"("Visible"=w1720) -> ()  [unwired: 2 in, 2 out]
        n1343 = property on="Port 4" class="Bool (strict)"("Visible"=w1720) -> ()  [unwired: 2 in, 2 out]
      }
      frame True {
        w1721 = TRUE ("Visible")
        n1344 = property on="Port 2a" class="Bool (strict)"("Visible"=w1721) -> ()  [unwired: 2 in, 2 out]
        n1345 = property on="Port 4" class="Bool (strict)"("Visible"=w1721) -> ()  [unwired: 2 in, 2 out]
      }
    }
    n1346 = Or(x=w1705, y="Re-initialize Port2") -> (x .or. y?=w1702:bool)
    n1347 = case shown="True" w1702 {
      tunnel: [w1716 errorcluster {"status"=TRUE, "code"=0, "source"="Init"} ("error out")] -> w1703
      tunnel: w1704 -> [w1716 _]
      frame False {
      }
      frame True {
      }
    }
    n1348 = case shown="No Error" w1703 {
      selector: w1703 -> [w1722 w1882]
      tunnel: [w1724 w1887] -> w1715
      tunnel: [w1723 w1880] -> w1714
      tunnel: w1706 -> [w1726 w1885]
      tunnel: [w1725 _] -> _
      frame No Error {
        n1349 = stacked-sequence {
          tunnel: w1726 -> [w1750 _]
          tunnel: w1722 -> [w1749 _]
          tunnel: [w1736 _] -> w1725
          tunnel: [w1735 _] -> w1724
          tunnel: [w1734 _] -> w1723
          frame #0 {
            n1350 = property class="Instr"(reference=w1750, error in=w1749) -> (reference out=w1733:refnum<visa-resource-name>, error out=w1748:errorcluster, "Serial Settings:Number of Bytes at Serial Port"=w1729:u32)
            "Port 2" <- w1729
            n1351 = Greater?(x=w1729, y=u32 23) -> (0:w1731:bool)
            n1352 = Not(x=w1731) -> ()  [unwired: 1 out]
            n1353 = case shown="True" w1731 {
              tunnel: w1733 -> [w1765 w1790]
              tunnel: w1748 -> [w1764 w1791]
              tunnel: [w1764 w1793] -> w1744
              tunnel: [w1765 w1792] -> w1745
              frame False {
              }
              frame True {
                # "Out as Volts"
                n1354 = local read "Residual Due"() -> (w1789:string)
                n1355 = while {
                  tunnel: [w1839] -> w1793
                  tunnel: [w1838] -> w1792
                  tunnel: w1791 -> [w1837]
                  tunnel: w1790 -> [w1836]
                  tunnel: [w1833] -> _
                  shift-right: [w1831] -> w1788
                  shift-left: w1789 -> [w1830]
                  i -> [w1833]
                  stop <- w1828 stop-if-true
                  n1356 = property class="Instr"(reference=w1836, error in=w1837) -> (reference out=w1841:refnum<visa-resource-name>, error out=w1840:errorcluster, "Serial Settings:Number of Bytes at Serial Port"=w1832:u32)
                  n1357 = local read "Quit"() -> (w1827:bool)
                  n1358 = VISA Read(VISA resource name=w1841, byte count=w1832, error in (no error)=w1840) -> (VISA resource name out=w1838:refnum<visa-resource-name>, read buffer=w1829:string, error out=w1839:errorcluster)  [unwired: 1 out]
                  n1359 = Greater?(x=w1832, y=u32 8) -> (0:w1834:bool)
                  n1360 = Compound Arithmetic op=OR(w1834, w1827) -> (w1828:bool)
                  n1361 = Concatenate Strings(w1830, w1829) -> (w1831:string)
                }
                n1362 = while {
                  shift-right: [w1820] -> w1772
                  shift-left: w1788 -> [w1825]
                  tunnel: [w1819] -> w1784 mode=indexing
                  tunnel: [w1818] -> _
                  i -> [w1818]
                  stop <- w1817 stop-if-true
                  n1363 = Match Pattern(string=w1825, regular expression="*") -> (after substring=w1823:string)  [unwired: 1 in, 3 out]
                  n1364 = local read "Quit"() -> (w1816:bool)
                  n1365 = Match Pattern(string=w1823, regular expression="&") -> (before substring=w1819:string, after substring=w1820:string, offset past match=w1821:i32)  [unwired: 1 in, 1 out]
                  n1366 = Less Than 0?(x=w1821) -> (x < 0?=w1822:bool)
                  n1367 = Compound Arithmetic op=OR(w1822, w1816) -> (w1817:bool)
                }
                n1368 = Array Size(array=w1784) -> (size(s)=w1787:i32)
                n1369 = local write "Residual Due"(w1772) -> ()
                n1370 = Decrement(x=w1787) -> (x-1=w1785:i32)
                n1371 = Delete From Array(array=w1784, length=1, index=w1785) -> (array with subset deleted=w1783:string[])  [unwired: 1 out]
                n1372 = Array Size(array=w1783) -> (size(s)=w1771:i32)
                n1373 = Decrement(x=w1771) -> (x-1=w1770:i32)
                n1374 = while {
                  tunnel: w1783 -> [w1804] mode=indexing
                  tunnel: w1770 -> [w1803]
                  tunnel: [w1801] -> w1778 mode=indexing
                  tunnel: [w1800] -> w1777 mode=indexing
                  tunnel: [w1799] -> w1776 mode=indexing
                  tunnel: [w1798] -> w1775 mode=indexing
                  tunnel: [w1797] -> w1773 mode=indexing
                  tunnel: [w1796] -> _
                  i -> [w1796]
                  stop <- w1795 stop-if-true
                  w1813 = u32 0 ("length (rest)")
                  w1812 = ";" ("regular expression")
                  n1375 = Less Or Equal?(x=w1803, y=w1796) -> (x <= y?=w1802:bool)
                  n1376 = Match Pattern(string=w1804, regular expression=w1812) -> (before substring=w1805:string, after substring=w1806:string)  [unwired: 1 in, 2 out]
                  n1377 = Match Pattern(string=w1806, regular expression=w1812) -> (before substring=w1809:string, after substring=w1807:string)  [unwired: 1 in, 2 out]
                  n1378 = local read "Quit"() -> (w1794:bool)
                  n1379 = Decimal String To Number(string=w1805, default (0L)=w1813) -> (number=w1801:u32)  [unwired: 1 in, 1 out]
                  n1380 = Decimal String To Number(string=w1809, default (0L)=w1813) -> (number=w1800:u32)  [unwired: 1 in, 1 out]
                  n1381 = Match Pattern(string=w1807, regular expression=w1812) -> (before substring=w1810:string, after substring=w1808:string)  [unwired: 1 in, 2 out]
                  n1382 = Decimal String To Number(string=w1810, default (0L)=w1813) -> (number=w1799:u32)  [unwired: 1 in, 1 out]
                  n1383 = Match Pattern(string=w1808, regular expression=w1812) -> (before substring=w1811:string, after substring=w1815:string)  [unwired: 1 in, 2 out]
                  n1384 = Compound Arithmetic op=OR(w1802, w1794) -> (w1795:bool)
                  n1385 = Decimal String To Number(string=w1811, default (0L)=w1813) -> (number=w1798:u32)  [unwired: 1 in, 1 out]
                  n1386 = Decimal String To Number(string=w1815, default (0L)=u8 0 ("length (rest)")) -> (number=w1797:u8)  [unwired: 1 in, 1 out]
                }
                "Din" <- w1773
                n1387 = Bundle(w1778, w1777, w1776, w1775) -> (w1780:cluster{u32[], u32[], u32[], u32[]})  [unwired: 1 in]
                n1388 = Divide(x=w1780, y=4095 ("length (rest)")) -> (x/y=w1782:cluster{dbl[], dbl[], dbl[], dbl[]})
                n1389 = Multiply(x=w1782, y=sgl 3.32 ("Numeric")) -> (x*y=w1774:cluster{dbl[], dbl[], dbl[], dbl[]})
                n1390 = Unbundle(w1774) -> (→"ECR":dbl[], →"Rtemp":dbl[], →"Air temp":dbl[], →"Ch3 2":dbl[])
              }
            }
            n1391 = call "Elapsed Time10"("Time Target (s)"=2.0, "Reset"=w1731, "Auto Reset"=FALSE) -> ("Time has Elapsed"=→"Port 2a":bool)  [unwired: 9 in, 7 out]
            n1392 = local read "Due Com"() -> (w1737:string[])
            n1393 = Array Size(array=w1737) -> (size(s)=w1736:i32)
            n1394 = Delete From Array(array=w1737, length=1, index=0) -> (deleted portion=w1740:string[], array with subset deleted=w1741:string[])
            n1395 = local write "Due Com"(w1741) -> ()
            n1396 = Index Array(array=w1740, index=0) -> (element=w1738:string)
            n1397 = Not Equal?(x=w1738, y="") -> (x != y?=w1746:bool)
            n1398 = case shown="True" w1746 {
              tunnel: w1745 -> [w1752 w1757]
              tunnel: [w1752 w1761] -> w1735
              tunnel: w1744 -> [w1751 w1756]
              tunnel: [w1751 w1759] -> w1734
              tunnel: w1738 -> [_ w1755]
              tunnel: [_ w1758] -> _
              frame False {
                # "DATA  WRITE LOOP"
              }
              frame True {
                n1399 = Concatenate Strings(w1755, "\r\n") -> (w1754:string)
                n1400 = VISA Write(VISA resource name=w1757, write buffer=w1754, error in (no error)=w1756) -> (VISA resource name out=w1761:refnum<visa-resource-name>, return count=w1758:u32, error out=w1760:errorcluster)
                n1401 = flat-sequence {
                  tunnel: w1760 -> [w1762]
                  tunnel: [w1762] -> w1759
                  frame #0 {
                    n1402 = Wait (ms)(milliseconds to wait=u32 5) -> ()  [unwired: 1 out]
                  }
                }
              }
            }
          }
          frame #1 {
            w1850 = 10 ("y")
            w1855 = 10 ("y")
            n1403 = local read "Rtemp"() -> (w1843:dbl[])
            n1404 = local read "ecr buf"() -> (w1844:dbl[])
            n1405 = for {
              tunnel: w1843 -> [w1867] mode=indexing
              shift-right: [w1868] -> w1851
              shift-left: dbl[] [] ("temp buf 2") -> [w1869]
              n1406 = Build Array (concatenate)(w1869, w1867) -> (w1870:dbl[])
              n1407 = Equal To 0?(x=w1867) -> (x = 0?=w1871:bool)
              n1408 = Select(t=w1869, s=w1871, f=w1870) -> (s? t:f=w1868:dbl[])
            }
            n1409 = local read "ECR"() -> (w1842:dbl[])
            n1410 = Insert Into Array(array=w1842, index=0, new element=w1844) -> (w1848:dbl[])
            n1411 = local read "temp buf"() -> (w1852:dbl[])
            n1412 = Array Size(array=w1848) -> (size(s)=w1849:i32)
            n1413 = Greater?(x=w1849, y=w1850) -> (0:w1847:bool)
            n1414 = case shown="True" w1847 {
              tunnel: w1848 -> [w1860 w1866]
              tunnel: w1849 -> [_ w1864]
              tunnel: w1850 -> [_ w1863]
              tunnel: [w1860 w1861] -> w1845
              frame False {
              }
              frame True {
                n1415 = Subtract(x=w1864, y=w1863) -> (x-y=w1862:i32)
                n1416 = Delete From Array(array=w1866, length=w1862, index=0) -> (array with subset deleted=w1861:dbl[])  [unwired: 1 out]
              }
            }
            "ecr buf" <- w1845
            n1417 = Insert Into Array(array=w1851, index=0, new element=w1852) -> (w1857:dbl[])
            n1418 = Array Size(array=w1857) -> (size(s)=w1856:i32)
            n1419 = Greater?(x=w1856, y=w1855) -> (0:w1858:bool)
            n1420 = case shown="True" w1858 {
              tunnel: w1857 -> [w1872 w1878]
              tunnel: w1856 -> [_ w1876]
              tunnel: w1855 -> [_ w1875]
              tunnel: [w1872 w1873] -> w1854
              frame False {
              }
              frame True {
                n1421 = Subtract(x=w1876, y=w1875) -> (x-y=w1874:i32)
                n1422 = Delete From Array(array=w1878, length=w1874, index=0) -> (array with subset deleted=w1873:dbl[])  [unwired: 1 out]
              }
            }
            "temp buf" <- w1854
          }
        }
      }
      frame Error {
        w1893 = u16 0 items=["None", "XON/XOFF", "RTS/CTS", "XON/XOFF & RTS/CTS", "DTR/DSR", "XON/XOFF & DTR/DSR"] ("flow control (0:none)  2")
        w1891 = u16 10 items=["1.0"=10, "1.5"=15, "2.0"=20] ("stop bits 2")
        w1889 = u16 0 items=["None", "Odd", "Even", "Mark", "Space"] ("parity 2")
        w1890 = u32 10000  # timeout (10sec)
        n1423 = VISA Clear(VISA resource name=w1885, error in (no error)=w1882) -> (VISA resource name out=w1884:refnum<visa-resource-name>, error out=w1883:errorcluster)
        n1424 = VISA Close(VISA resource name=w1884, error in (no error)=w1883) -> (error out=w1886:errorcluster)
        n1425 = call <vilib>:"Clear Errors.vi"("error in (no error)"=w1886) -> ()  [unwired: 5 in, 2 out]
        n1426 = local read "Com Port 2"() -> (w1879:refnum<visa-resource-name>)
        "visa due" <- w1879
        n1427 = call-poly "VISA Configure Serial Port"("VISA resource name"=w1879, "timeout (10sec)"=w1890, "baud rate (9600)"=u32 250000 ("baud rate  2"), "data bits (8)"=u16 8 ("data bits  2"), "parity (0:none)"=w1889, "stop bits (10: 1 bit)"=w1891, "flow control (0:none)"=w1893) -> ("VISA resource name out"=w1894:refnum<visa-resource-name>, "error out"=w1895:errorcluster)  [unwired: 7 in]
        n1428 = flat-sequence {
          tunnel: w1894 -> [w1897]
          tunnel: w1895 -> [w1896]
          tunnel: [w1897] -> w1887
          tunnel: [w1896] -> w1880
          frame #0 {
            n1429 = Wait (ms)(milliseconds to wait=u32 50) -> ()  [unwired: 1 out]
          }
        }
        "Residual Due" <- ""
        "Port 2 Error" <- w1880
      }
    }
    n1430 = local read "Quit"() -> (w1701:bool)
    "Error Due" <- w1708
  }
  n1431 = property on="RUN" class="Bool (strict)"("Visible"=TRUE) -> ()  [unwired: 2 in, 2 out]
  n1432 = while {
    tunnel: [w1915] -> _
    tunnel: [w1899] -> w55
    i -> [w1915]
    stop <- w1899 stop-if-true
    n1433 = local read "conststatus"() -> (w1903:dbl)
    n1434 = local read "Main Tab"() -> (w1901:T2)
    n1435 = local read "EDIT"() -> (w1921:bool)
    n1436 = local read "Rate"() -> (w1920:dbl)
    n1437 = case shown="True" w1921 {
      tunnel: [FALSE TRUE] -> w1907
      frame False {
      }
      frame True {
      }
    }
    n1438 = property on="Time slide" class="Slide (strict)"("Scale.Range:Maximum"=2500.0) -> ()  [unwired: 2 in, 2 out]
    n1439 = Equal?(x=w1901, y=T23."About" ("Main Tab")) -> (x = y?=w1913:bool)
    n1440 = Equal?(x=w1903, y=0.0) -> (x = y?=w1904:bool)
    n1441 = Divide(x=1.0, y=w1920) -> (x/y=w1916:dbl)
    "Time 2" <- w1916
    n1442 = case shown="True" w1904 {
      frame False {
      }
      frame True {
        # "C:\\WinDucom\\calibrate WO 2391.dcf"
        n1443 = local write "Lan flag"(22) -> ()
        n1444 = local write "conststatus"(10.0 ("rpm value : 2")) -> ()
        n1445 = String To Path(string="C:\\LAB-IQ\\calibrate WO 2465.dcf") -> (path=w1927:path)
        n1446 = Open/Create/Replace File "Open File"(file path (use dialog)=w1927) -> (refnum out=w1925:refnum<file>)  [unwired: 5 in, 2 out]
        n1447 = for {
          N: 23 -> [_]
          tunnel: w1925 -> [w1936]
          i -> [w1930]
          (unwired) TRUE ("line mode (F)")
          n1448 = Read from Text File "Read File"(file (use dialog)=w1936) -> (text=w1935:string)  [unwired: 3 in, 3 out]
          n1449 = Match Pattern(string=w1935, regular expression="]") -> (after substring=w1933:string)  [unwired: 1 in, 3 out]
          n1450 = String Subset(string=w1935, offset (0)=5, length (rest)=10 ("length (rest)")) -> (substring=w1928:string)
          n1451 = Fract/Exp String To Number(string=w1928) -> (number=w1929:dbl)  [unwired: 3 in, 1 out]
          n1452 = Match Pattern(string=w1933, regular expression="-") -> (before substring=w1931:string)  [unwired: 1 in, 3 out]
          n1453 = case shown="8" w1930 {
            tunnel: w1929 -> [w1939 w1940 w1941 w1942 _ _ _ w1947 w1948 w1949 w1952 w1953 w1954 w1955 w1956 w1957 w1958 w1961 w1962 _ _ w1965 _ _]
            tunnel: w1931 -> [_ _ _ _ w1943 w1944 w1945 _ _ _ _ _ _ _ _ _ _ _ _ w1963 w1964 _ w1966 _]
            frame 0 {
              n1454 = local write "FRIC. FORCE :"(w1939) -> ()
            }
            frame 1 {
              n1455 = local write "TEMPERATURE :"(w1940) -> ()
            }
            frame 2 {
              n1456 = local write "HUMIDITY:"(w1941) -> ()
            }
            frame 3 {
              n1457 = local write "AIR TEMPERATURE :"(w1942) -> ()
            }
            frame 4 {
              n1458 = local write "Com Port 1"(w1943) -> ()
            }
            frame 5 {
              n1459 = local write "Com Port 2"(w1944) -> ()
              n1460 = local write "visa due"(w1944) -> ()
            }
            frame 6 {
              n1461 = String To Path(string=w1945) -> (path=w1946:path)
              n1462 = local write "File Path"(w1946) -> ()
              "String" <- w1945
            }
            frame 7 {
              n1463 = local write "DISPLACEMENT :"(w1947) -> ()
            }
            frame 8 {
              n1464 = local write "STROKE GAIN :"(w1948) -> ()
            }
            frame 9 {
              n1465 = local read "Stroke PID Gains"() -> (w1951:T9)
              n1466 = Bundle By Name(cluster=w1951, "Proportional Gain (Kc)"=w1949) -> (w1950:T9)
              n1467 = local write "Stroke PID Gains"(w1950) -> ()
            }
            frame 10 {
              n1468 = local write "Language Selection"(w1952) -> ()
            }
            frame 11 {
              n1469 = local write "CH-POWER +"(w1953) -> ()
            }
            frame 12 {
              n1470 = local write "CH-POWER -"(w1954) -> ()
            }
            frame 13 {
              n1471 = local write "CH-HEATER"(w1955) -> ()
            }
            frame 14 {
              n1472 = local write "CH-HUMIDITY WET"(w1956) -> ()
            }
            frame 15 {
              n1473 = local write "CH-HUMIDITY DRY"(w1957) -> ()
            }
            frame 16 {
              n1474 = local read "Stroke PID Gains"() -> (w1960:T9)
              n1475 = Bundle By Name(cluster=w1960, "Integral Time (Ti, min)"=w1958) -> (w1959:T9)
              n1476 = local write "Stroke PID Gains"(w1959) -> ()
            }
            frame 17 {
              n1477 = local write "AIR TEMP INTERCEPT:"(w1961) -> ()
            }
            frame 18 {
              n1478 = local write "TEMP INTERCEPT:"(w1962) -> ()
            }
            frame 19 {
              n1479 = local write "S.NO"(w1963) -> ()
            }
            frame 20 {
              n1480 = local write "Com Port 3"(w1964) -> ()
            }
            frame 21 {
              n1481 = local write "LvdtOff"(w1965) -> ()
            }
            frame 22 {
              n1482 = local write "C3 :"(w1966) -> ()
            }
            frame 23, Default {
            }
          }
        }
      }
    }
    n1483 = Select(t=u32 2500 ("milliseconds to wait"), s=w1913, f=u32 500 ("milliseconds to wait")) -> (s? t:f=w1911:u32)
    n1484 = Multiply(x=w1916, y=w1911) -> (x*y=w1918:dbl)
    n1485 = property on="FF Calibration g" class="WFGraph (strict)"("Visible"=w1907) -> ()  [unwired: 2 in, 2 out]
    n1486 = property on="Lift" class="Bool (strict)"("Visible"=w1907) -> ()  [unwired: 2 in, 2 out]
    n1487 = property on="Threshold" class="DigNum (strict)"("Visible"=w1907) -> ()  [unwired: 2 in, 2 out]
    n1488 = property on="Time slide" class="Slide (strict)"("Visible"=w1907) -> ()  [unwired: 2 in, 2 out]
    n1489 = call "Elapsed Time2"("Time Target (s)"=w1918, "Auto Reset"=TRUE) -> ("Time has Elapsed"=w1908:bool)  [unwired: 10 in, 7 out]
    n1490 = case shown="True" w1908 {
      frame False {
        # "79.77669138"
        # "2.3554"
        n1491 = local read "FRIC. FORCE :"() -> (w1971:dbl)
        n1492 = local read "FF cal val"() -> (w1968:dbl[])
        n1493 = Multiply(x=w1971, y=79.77669138) -> (x*y=w1970:dbl)
        n1494 = Multiply(x=w1968, y=w1970) -> (x*y=→"FF Calibration g":dbl[])
        "Err Count" <- 0 ("y")
      }
      frame True {
        n1495 = stacked-sequence {
          frame #0 {
            n1496 = stacked-sequence {
              frame #0 {
                "Lift" <- TRUE ("Lift")
              }
            }
          }
          frame #1 {
            w1983 = 2500 ("y")
            n1497 = local read "RUN"() -> (w1975:bool)
            n1498 = local read "FF1"() -> (w1978:dbl[])
            n1499 = case shown="False" w1975 {
              frame False {
                n1500 = local write "Frequency"(0.0 ("Frequency")) -> ()
              }
              frame True {
              }
            }
            n1501 = Array Size(array=w1978) -> (size(s)=w1977:i32)
            n1502 = local read "Ch1"() -> (w1974:dbl[])
            "Waveform Chart 2" <- w1974
            n1503 = call-poly <vilib>:"Mean.vi"("X"=w1974) -> ("mean"=→"Raw Mean":dbl)  [unwired: 1 out]
            n1504 = Insert Into Array(array=w1978, index=w1977, new element=w1974) -> (w1980:dbl[])
            n1505 = Array Size(array=w1980) -> (size(s)=w1984:i32)
            n1506 = Subtract(x=w1984, y=w1983) -> (x-y=w1982:i32)
            n1507 = Greater?(x=w1984, y=w1983) -> (0:w1985:bool)
            n1508 = case shown="True" w1985 {
              tunnel: w1982 -> [_ w1989]
              tunnel: [w1987 w1991] -> w1976
              tunnel: w1980 -> [w1987 w1990]
              frame False {
              }
              frame True {
                n1509 = Delete From Array(array=w1990, length=w1989, index=0) -> (array with subset deleted=w1991:dbl[])  [unwired: 1 out]
                "Numeric" <- w1989
              }
            }
            "FF1" <- w1976
            "PID Ref" <- TRUE ("PID Ref")
          }
          frame #2 {
          }
          frame #3 {
            # "CONVERT TO N"
            # "DATA PROCESSING"
            # "115 mV/N"
            n1510 = local read "RH Numeric:"() -> (w1997:dbl)
            n1511 = local read "HUMIDITY:"() -> (w1998:dbl)
            n1512 = local read "temp buf"() -> (w2059:dbl[])
            n1513 = local read "Air temp"() -> (w2057:dbl[])
            n1514 = local read "ecr buf"() -> (w2019:dbl[])
            n1515 = local read "Fric Val"() -> (w2062:dbl[])
            n1516 = case shown="True" "Reset Button" {
              frame False {
              }
              frame True {
                n1517 = local write "Reset Button"(FALSE) -> ()
                n1518 = local write "Captured Values"(dbl[][] [] ("Captured Values")) -> ()
                n1519 = local write "Best Fit"(dbl[] [] ("Best Fit")) -> ()
              }
            }
            n1520 = local read "TEMPERATURE :"() -> (w2040:dbl)
            n1521 = call-poly <vilib>:"Mean.vi"("X"=w2019) -> ("mean"=w2016:dbl)  [unwired: 1 out]
            n1522 = call-poly <vilib>:"Mean.vi"("X"=w2057) -> ("mean"=w2026:dbl)  [unwired: 1 out]
            "Raw air temp" <- w2026
            n1523 = call-poly <vilib>:"Mean.vi"("X"=w2059) -> ("mean"=w2028:dbl)  [unwired: 1 out]
            "Raw specimen temp" <- w2028
            n1524 = local read "TEMP INTERCEPT:"() -> (w2033:dbl)
            n1525 = Multiply(x=w1997, y=w1998) -> (x*y=→"Humidity ( %RH )" →"Hum" →"Hum 2":dbl)
            n1526 = Multiply(x=w2062, y=1.0) -> (x*y=w2063:dbl[])
            n1527 = local read "FRIC. FORCE :"() -> (w2056:dbl)
            n1528 = Multiply(x=w2028, y=w2040) -> (x*y=w2022:dbl)
            n1529 = local read "AIR TEMPERATURE :"() -> (w2041:dbl)
            n1530 = local read "RUN"() -> (w2053:bool)
            n1531 = Add(x=w2026, y="Offset Air Temp") -> (x+y=w2021:dbl)
